vi "Is_Linux_Target.vi"(8 "error in (no error)":errorcluster, 10 "buildObject":T1, 11 "AB_Build in":refnum<class "AB_Build.lvclass">) -> (0 "error out":errorcluster, 2 "Linux?":bool, 3 "AB_Build out":refnum<class "AB_Build.lvclass">)   [LabVIEW 2020, in "AB_Build.lvclass"]
uses:
  <vilib>/AppBuilder/AB_Classes/Build/AB_Build.lvclass
  <vilib>/AppBuilder/AB_Classes/Build/AB_Build.lvclass/AB_Build.ctl
  <resource>/Framework/Providers/API/ItemRef.ctl
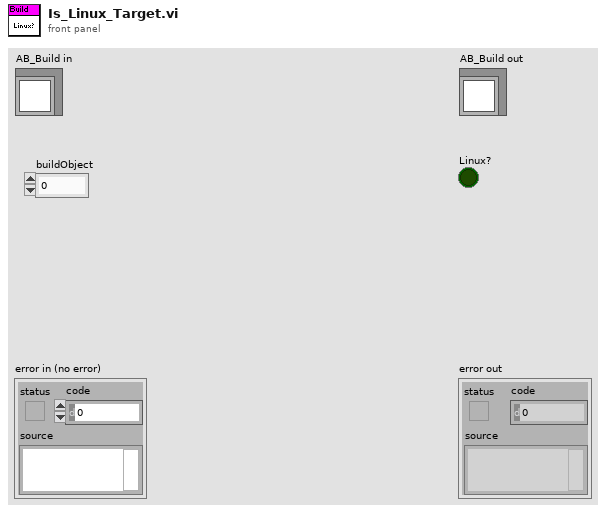
[diagram p1: front panel]
types:
  T1 = typedef "ItemRef.ctl" = u64
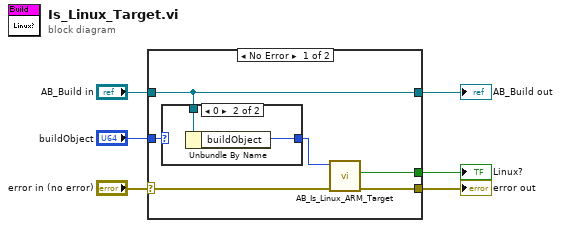
[diagram p0: block diagram]
diagram:
  n1 = case shown="No Error" "error in (no error)" {
    selector: "error in (no error)" -> [w9 w17]
    tunnel: [w8 w17] -> w5
    tunnel: [w12 w16] -> w3
    tunnel: "AB_Build in" -> [w12 w16]
    tunnel: [w7 _] -> w2
    tunnel: "buildObject" -> [w11 _]
    frame No Error {
      n2 = case shown="0" w11 {
        selector: w11 -> [w13 _]
        tunnel: [w13 w15] -> w10
        tunnel: w12 -> [_ w14]
        frame Default {
        }
        frame 0 {
          n3 = Unbundle By Name(w14) -> ("buildObject"=w15:T1)
        }
      }
      n4 = call <resource>:"AB_Is_Linux_ARM_Target.vi"("error in (no error)"=w9, "Object"=w10) -> ("error out"=w8:errorcluster, "Linux target?"=w7:bool)  [unwired: 7 in, 1 out]
    }
    frame Error {
    }
  }
  "error out" <- w5
  "AB_Build out" <- w3
  "Linux?" <- w2
